vi "CountTrialOutcomes.vi"(11 "Mouse Performance in":i16[][](array[numeric])) -> (0 "nFalseAlarms":i32, 1 "nMiss":i32, 2 "nCorrect Rejections":i32, 3 "nHits":i32, 4 "nGoTrials":i16, 5 "nTrials":i32)   [LabVIEW 2013]
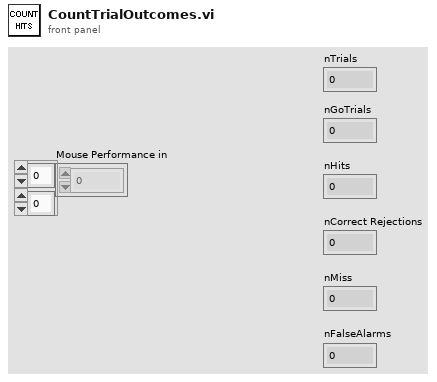
[diagram p1: front panel]
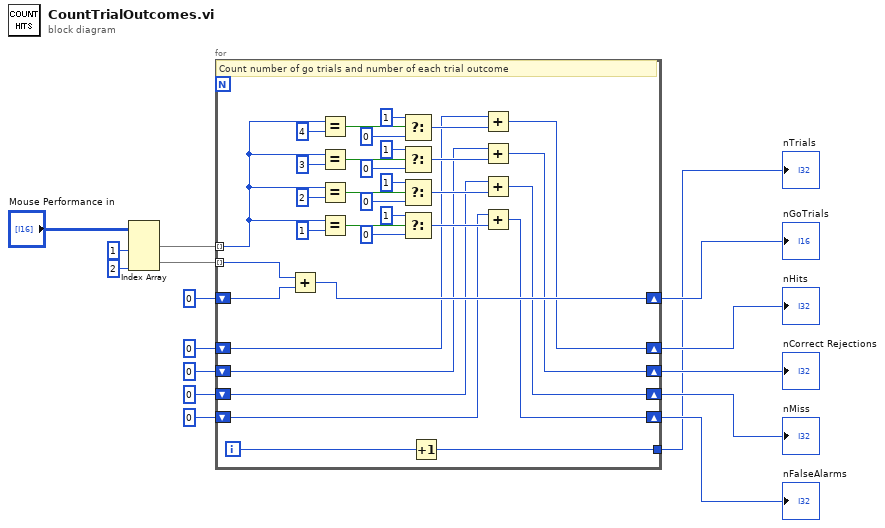
[diagram p0: block diagram]
diagram:
  n1 = Index Array(array="Mouse Performance in", index (col) #1=1 ("disabled index (col)"), index (col) #2=2 ("index (col)")) -> (element #1=w13:i16[], element #2=w12:i16[])  [unwired: 2 in]
  n2 = for {
    tunnel: w13 -> [w47] mode=indexing
    tunnel: w12 -> [w50] mode=indexing
    shift-right: [w48] -> w6
    shift-left: i16 0 -> [w49]
    shift-right: [w22] -> w2
    shift-left: 0 -> [w23]
    shift-right: [w21] -> w3
    shift-left: 0 -> [w24]
    shift-right: [w20] -> w4
    shift-left: 0 -> [w25]
    shift-right: [w19] -> w5
    shift-left: 0 -> [w26]
    tunnel: [w17] -> w1
    i -> [w18]
    # "Count number of go trials and number of each trial outcome"
    n3 = Add(x=w50, y=w49) -> (x+y=w48:i16)
    n4 = Equal?(x=w47, y=i16 4) -> (x = y?=w42:bool)
    n5 = Equal?(x=w47, y=i16 3) -> (x = y?=w40:bool)
    n6 = Equal?(x=w47, y=i16 2) -> (x = y?=w39:bool)
    n7 = Equal?(x=w47, y=i16 1) -> (x = y?=w41:bool)
    n8 = Select(t=1, s=w42, f=0) -> (s? t:f=w30:i32)
    n9 = Select(t=1, s=w40, f=0) -> (s? t:f=w29:i32)
    n10 = Select(t=1, s=w39, f=0) -> (s? t:f=w28:i32)
    n11 = Select(t=1, s=w41, f=0) -> (s? t:f=w27:i32)
    n12 = Increment(x=w18) -> (x+1=w17:i32)
    n13 = Add(x=w26, y=w30) -> (x+y=w19:i32)
    n14 = Add(x=w25, y=w29) -> (x+y=w20:i32)
    n15 = Add(x=w24, y=w28) -> (x+y=w21:i32)
    n16 = Add(x=w23, y=w27) -> (x+y=w22:i32)
  }
  "nGoTrials" <- w6
  "nHits" <- w5
  "nCorrect Rejections" <- w4
  "nMiss" <- w3
  "nFalseAlarms" <- w2
  "nTrials" <- w1
